vi "Globals.vi"() -> ()   [LabVIEW 2016]
panel:
  in  "Inventory File Path Windows":path=path "C:/Users/hsallim/Desktop/Inventory Test.xml"
  in  "Inventory File Path RT":path=path "c:/ni-rt/Inventory/Inventory.xml"
  in  "Inventory File Path":path=path "c:/ni-rt/Inventory/Inventory.xml"
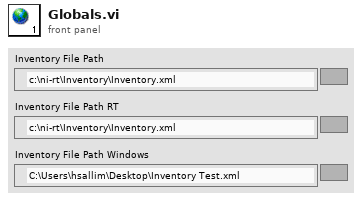
[diagram p1: front panel]
diagram:
